vi "Focus_Z_calc.vi"(7 "KinfeThickness":dbl caption="Kinfe Edge Total Thickness", 10 "FocusPos.":dbl, 11 "SampleThickness":dbl caption="Sample Total Thickness") -> (2 "Z":dbl)   [LabVIEW 2011]
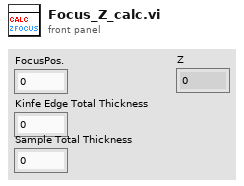
[diagram p1: front panel]
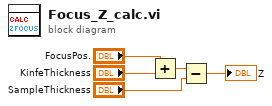
[diagram p0: block diagram]
diagram:
  n1 = Add(x="FocusPos.", y="KinfeThickness") -> (x+y=w2:dbl)
  n2 = Subtract(x=w2, y="SampleThickness") -> (x-y=→"Z":dbl)
